vi "Get Status.vi"(11 "Plugin in":refnum<class "Plugin.lvclass">) -> (2 "status pointer":refnum<class "Status Pointer.lvclass">, 3 "Plugin out":refnum<class "Plugin.lvclass">)   [LabVIEW 2021, in "DSF Core.lvlib" / "Plugin.lvclass"]
uses:
  Plugin.lvclass
  Status/Status Pointer.lvclass
  Plugin.lvclass/Plugin.ctl
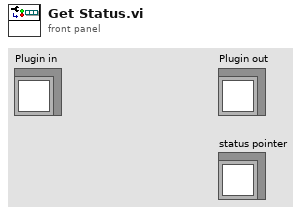
[diagram p1: front panel]
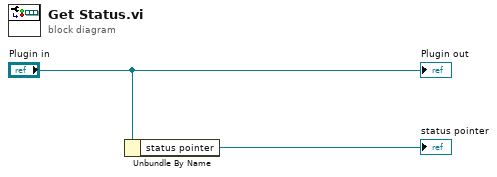
[diagram p0: block diagram]
diagram:
  n1 = Unbundle By Name("Plugin in") -> ("status pointer"=→"status pointer":refnum<class "Status Pointer.lvclass">)
  "Plugin out" <- "Plugin in"
